vi "Teleop Roller.vi"(10 "Roller Speed":dbl, 11 "Joystick Data":T1) -> ()   [LabVIEW 2013]
uses:
  Joystick Data.ctl
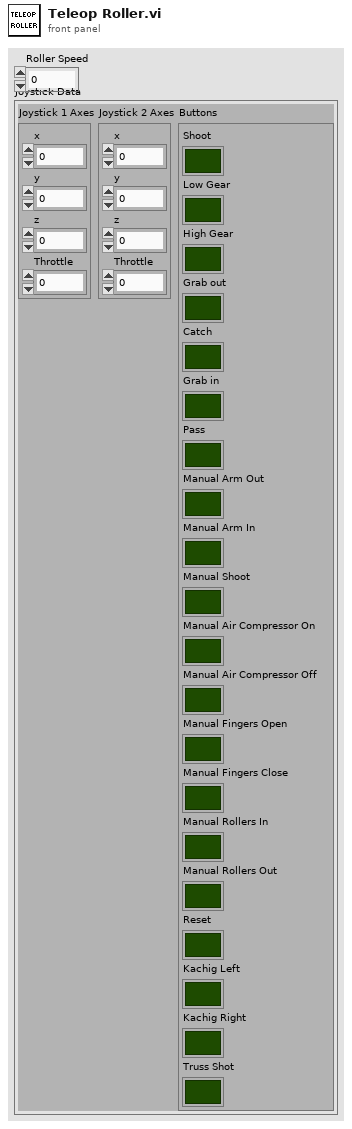
[diagram p1: front panel]
types:
  T1 = typedef "Joystick Data.ctl" = cluster{"Joystick 1 Axes":cluster{"x":dbl, "y":dbl, "z":dbl, "Throttle":dbl}, "Joystick 2 Axes":cluster{"x":dbl, "y":dbl, "z":dbl, "Throttle":dbl}, "Buttons":cluster{"Shoot":bool, "Low Gear":bool, "High Gear":bool, "Grab out":bool, "Catch":bool, "Grab in":bool, "Pass":bool, "Manual Arm Out":bool, "Manual Arm In":bool, "Manual Shoot":bool, "Manual Air Compressor On":bool, "Manual Air Compressor Off":bool, "Manual Fingers Open":bool, "Manual Fingers Close":bool, "Manual Rollers In":bool, "Manual Rollers Out":bool, "Reset":bool, "Kachig Left":bool, "Kachig Right":bool, "Truss Shot":bool}}
  T2 = typedef "WPI_MotorControlDeviceRef.ctl" = cluster{"DeviceStatus":errorcluster, "Type":enum16{"PWM", "CAN"}, "PWM":cluster{"Digital Module":T3, "PWM Channel":T4, "DeadBand":T5}, "CAN":cluster{"Device Number":u8, "Control Mode":T6, "Semaphore":T7, "Max Vout":dbl}, "Invert":bool, "TransformRef":T8, "InvTransformRef":T8}
  T3 = typedef "FPGA_TypedefDigitalModule.ctl" = enum16{"Digital Module 1", "Digital Module 2"}
  T4 = typedef "FPGA_DIOPWMChannel.ctl" = enum8{"PWM 1", "PWM 2", "PWM 3", "PWM 4", "PWM 5", "PWM 6", "PWM 7", "PWM 8", "PWM 9", "PWM 10", "Invalid"}
  T5 = typedef "WPI_PWMDeadband.ctl" = cluster{"Name":string, "maxPositivePwm":i32, "minPositivePwm":i32, "centerPwm":i32, "maxNegativePwm":i32, "minNegativePwm":i32, "angularRange":u16}
  T6 = typedef "WPI_CANJaguar_ControlMode.ctl" = enum8{"Percent VBus", "Current", "Speed", "Position", "Voltage"}
  T7 = typedef "Semaphore RefNum" = refnum<k1>
  T8 = typedef "WPI_PWMTransform_ConPane.ctl" = refnum<vi>
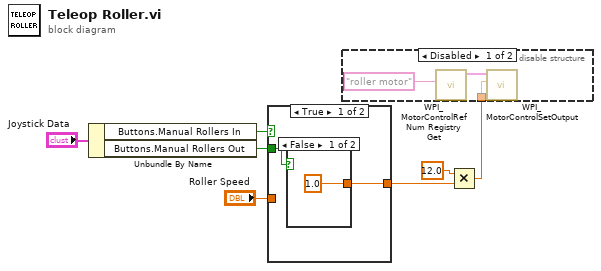
[diagram p0: block diagram]
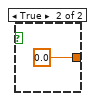
[diagram p3: hidden frame]
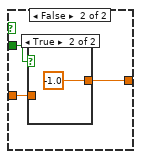
[diagram p4: hidden frame]
diagram:
  n1 = Unbundle By Name("Joystick Data") -> ("Buttons.Manual Rollers In"=w5:bool, "Buttons.Manual Rollers Out"=w4:bool)
  n2 = case shown="True" w5 {
    tunnel: w4 -> [w9 w14]
    tunnel: [w8 w13] -> w2
    tunnel: "Roller Speed" -> [_ w12]
    frame True {
      n3 = case shown="False" w9 {
        tunnel: [1.0 0.0] -> w8
        frame False {
        }
        frame True {
        }
      }
    }
    frame False {
      n4 = case shown="True" w14 {
        tunnel: [w15 -1.0] -> w13
        tunnel: w12 -> [w15 _]
        frame False {
        }
        frame True {
        }
      }
    }
  }
  n5 = Multiply(x=12.0, y=w2) -> (x*y=w3:dbl)
  n6 = disable-structure shown="Disabled" {
    disable-tunnel: w3 -> [w17 _]
    frame Disabled {
      n7 = call <vilib>:"WPI_MotorControlRefNum Registry Get.vi"("refnum name"="roller motor") -> ("MotorControlDevRef"=w18:T2)  [unwired: 9 in, 1 out]
      n8 = call <vilib>:"WPI_MotorControlSetOutput.vi"("Output"=w17, "MotorControlDevRef"=w18) -> ()  [unwired: 7 in, 3 out]
    }
    frame Enabled {
    }
  }
